vi "Table Test.vi"() -> ()   [LabVIEW 2012]
uses:
  Type/_Table Type.ctl
  Type/_RT Command.ctl
  Configuration/_Global Configuration.vi
panel:
  out "Max Index New":i32
  out "Max Diff New":i32
  out "Current step":i32
  in  "Start":bool
  in  "Table Type":T1
  out "Array":i32[][](array[numeric])
  out "Max Index Old":i32
  out "# of Steps":u32
  out "Max Diff Old":i32
  in  "Step Mass":dbl=0.1
  in  "Stop Mass":dbl=100.0
  in  "Start Mass":dbl
  # "New DAC"
  # "Old DAC"
  # "Actual DAC"
  # "Mass (1/100 amu)"
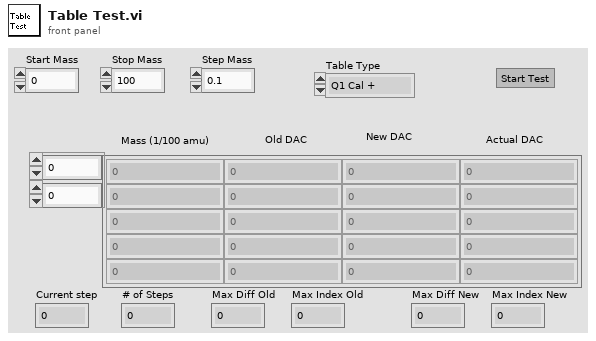
[diagram p1: front panel]
types:
  T1 = typedef "_Table Type.ctl" = enum8{"Q1 Cal +", "Q2 Cal +", "Q1 Cal -", "Q2 Cal -", "Q1 Res Hi +", "Q2 Res Hi +", "Q1 Res Med +", "Q2 Res Med +", "Q1 Res Lo +", "Q2 Res Lo +", "Q1 Res Hi -", "Q2 Res Hi -", "Q1 Res Med -", "Q2 Res Med -", "Q1 Res Lo -", "Q2 Res Lo -"}
  T2 = typedef "_RT Command.ctl" = enum16{"Start", "Stop", "Runtime Update", "Get Data", "Get Info", "Get Status", "Get Param", "Get Config", "Get Table", "Read ADC", "Set Oscillator", "Update Config", "Update Table", "Set All Pol", "Set Pol and DC", "Set Max Mass", "Toggle RP", "Toggle EL", "Set PIC", "Initialize Turbo", "Send Turbo Comm", "Close Turbo", "P1", "P2", "P3", "Send Serial", "Set LC Out", "Get LC In", "Read VAC", "Test Table", "Toggle Power", "Get Startup", "Set Startup", "Get ADC Table", "Set ADC Table", "Get Brief Status", "Get Detail Status", "Auxiliary Update", "Set CC Logics", "Set CC Input Logics", "Ignore Error"}
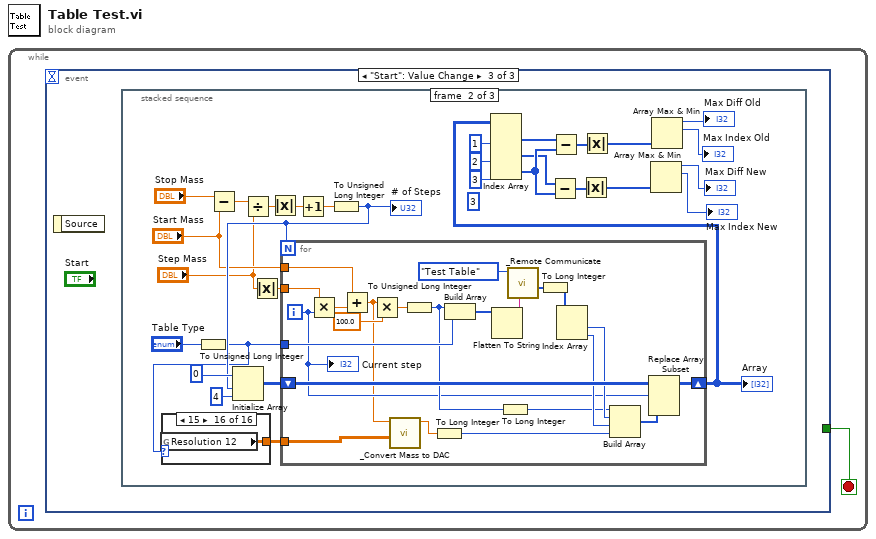
[diagram p0: block diagram]
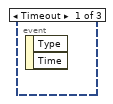
[diagram p2: hidden frame]
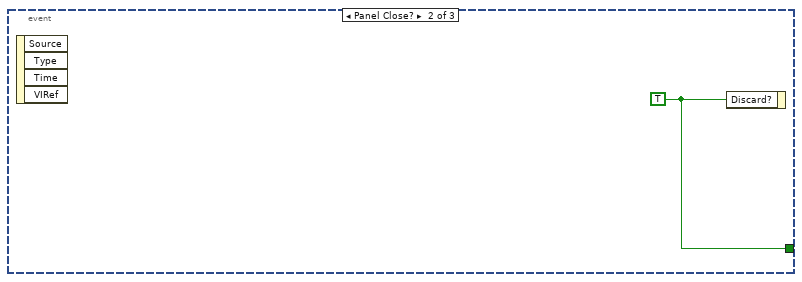
[diagram p3: hidden frame]
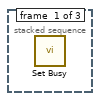
[diagram p4: hidden frame]
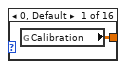
[diagram p5: hidden frame]
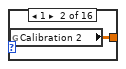
[diagram p6: hidden frame]
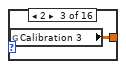
[diagram p7: hidden frame]
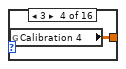
[diagram p8: hidden frame]
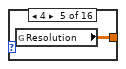
[diagram p9: hidden frame]
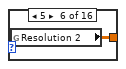
[diagram p10: hidden frame]
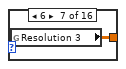
[diagram p11: hidden frame]
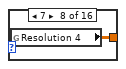
[diagram p12: hidden frame]
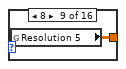
[diagram p13: hidden frame]
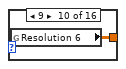
[diagram p14: hidden frame]
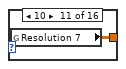
[diagram p15: hidden frame]
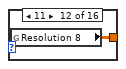
[diagram p16: hidden frame]
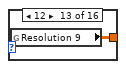
[diagram p17: hidden frame]
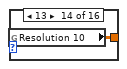
[diagram p18: hidden frame]
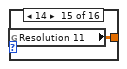
[diagram p19: hidden frame]
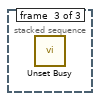
[diagram p20: hidden frame]
diagram:
  n1 = while {
    stop <- w1 stop-if-true
    n2 = event shown="[2] \"Start\": Value Change" {
      selector: _ -> [_ _ _]
      dyn-events: _ -> [_ _ _]
      timeout: _ -> [_ _ _]
      tunnel: [_ w2 _] -> w1
      event Timeout {
        n3 = event-data() -> ()  [unwired: 3 out]
      }
      event Panel Close? {
        w2 = TRUE ("Discard?")
        n4 = event-data() -> ()  [unwired: 5 out]
        n5 = event-data("Discard?"=w2) -> ()  [unwired: 1 in, 1 out]
      }
      event "Start": Value Change {
        n6 = event-data() -> ()  [unwired: 2 out]
        n7 = stacked-sequence {
          frame #0 {
            n8 = call <vilib>:"Set Busy.vi"() -> ()  [unwired: 4 in, 8 out]
          }
          frame #1 {
            (unwired) 3 ("disabled index (col)")
            n9 = To Unsigned Long Integer(number="Table Type") -> (unsigned 32bit integer=w16:u32)
            n10 = case shown="15" w16 {
              tunnel: [w33 w34 w35 w36 w37 w38 w39 w40 w41 w42 w43 w44 w45 w46 w47 w48] -> w15
              frame 0, Default {
                n11 = global read "_Global Configuration.vi" "Calibration"() -> (w33:dbl[][])
              }
              frame 1 {
                n12 = global read "_Global Configuration.vi" "Calibration 2"() -> (w34:dbl[][])
              }
              frame 2 {
                n13 = global read "_Global Configuration.vi" "Calibration 3"() -> (w35:dbl[][])
              }
              frame 3 {
                n14 = global read "_Global Configuration.vi" "Calibration 4"() -> (w36:dbl[][])
              }
              frame 4 {
                n15 = global read "_Global Configuration.vi" "Resolution"() -> (w37:dbl[][])
              }
              frame 5 {
                n16 = global read "_Global Configuration.vi" "Resolution 2"() -> (w38:dbl[][])
              }
              frame 6 {
                n17 = global read "_Global Configuration.vi" "Resolution 3"() -> (w39:dbl[][])
              }
              frame 7 {
                n18 = global read "_Global Configuration.vi" "Resolution 4"() -> (w40:dbl[][])
              }
              frame 8 {
                n19 = global read "_Global Configuration.vi" "Resolution 5"() -> (w41:dbl[][])
              }
              frame 9 {
                n20 = global read "_Global Configuration.vi" "Resolution 6"() -> (w42:dbl[][])
              }
              frame 10 {
                n21 = global read "_Global Configuration.vi" "Resolution 7"() -> (w43:dbl[][])
              }
              frame 11 {
                n22 = global read "_Global Configuration.vi" "Resolution 8"() -> (w44:dbl[][])
              }
              frame 12 {
                n23 = global read "_Global Configuration.vi" "Resolution 9"() -> (w45:dbl[][])
              }
              frame 13 {
                n24 = global read "_Global Configuration.vi" "Resolution 10"() -> (w46:dbl[][])
              }
              frame 14 {
                n25 = global read "_Global Configuration.vi" "Resolution 11"() -> (w47:dbl[][])
              }
              frame 15 {
                n26 = global read "_Global Configuration.vi" "Resolution 12"() -> (w48:dbl[][])
              }
            }
            n27 = Subtract(x="Stop Mass", y="Start Mass") -> (x-y=w31:dbl)
            n28 = Divide(x=w31, y="Step Mass") -> (x/y=w29:dbl)
            n29 = Absolute Value(x="Step Mass") -> (abs(x)=w21:dbl)
            n30 = Absolute Value(x=w29) -> (abs(x)=w30:dbl)
            n31 = Increment(x=w30) -> (x+1=w28:dbl)
            n32 = To Unsigned Long Integer(number=w28) -> (unsigned 32bit integer=w26:u32)
            "# of Steps" <- w26
            n33 = Initialize Array(0, w26, 4 ("dimension size")) -> (w24:i32[][])
            n34 = for {
              N: w26 -> [_]
              shift-right: [w61] -> w19
              shift-left: w24 -> [w62]
              tunnel: "Start Mass" -> [w69]
              tunnel: w21 -> [w71]
              tunnel: w16 -> [w67]
              tunnel: w15 -> [w53]
              i -> [w56]
              n35 = Multiply(x=w71, y=w56) -> (x*y=w70:dbl)
              n36 = Add(x=w69, y=w70) -> (x+y=w54:dbl)
              n37 = Multiply(x=w54, y=100.0) -> (x*y=w55:dbl)
              n38 = call "_Convert Mass to DAC.vi"("Calibration Table"=w53, "Mass"=w54) -> ("DAC Value"=w52:dbl)  [unwired: 2 in, 3 out]
              n39 = To Unsigned Long Integer(number=w55) -> (unsigned 32bit integer=w60:u32)
              n40 = To Long Integer(number=w52) -> (32bit integer=w51:i32)
              n41 = Build Array(w60, w67) -> (w66:u32[])
              n42 = Flatten To String(anything=w66) -> (data string=w65:string)  [unwired: 1 in, 4 out]
              n43 = To Long Integer(number=w60) -> (32bit integer=w50:i32)
              n44 = call "_Remote Communicate.vi"("String"=w65, "Command"=_RT_Command."Test Table") -> ("Data Array"=w63:i32[])  [unwired: 4 in, 3 out]
              n45 = To Long Integer(number=w63) -> (32bit integer=w49:i32[])
              n46 = Index Array(array=w49) -> (element #1=w59:i32, element #2=w58:i32)  [unwired: 2 in]
              n47 = Build Array(w50, w59, w58, w51) -> (w57:i32[])
              n48 = Replace Array Subset(array=w62, new element=w57, index (row)=w56) -> (w61:i32[][])  [unwired: 1 in]
              "Current step" <- w56
            }
            "Array" <- w19
            n49 = Index Array(array=w19, index (col) #1=1 ("disabled index (col)"), index (col) #2=2 ("index (col)"), index (col) #3=3 ("index (col)")) -> (element #1=w11:i32[], element #2=w5:i32[], element #3=w6:i32[])  [unwired: 3 in]
            n50 = Subtract(x=w5, y=w6) -> (x-y=w7:i32[])
            n51 = Subtract(x=w11, y=w6) -> (x-y=w10:i32[])
            n52 = Absolute Value(x=w7) -> (abs(x)=w8:i32[])
            n53 = Absolute Value(x=w10) -> (abs(x)=w9:i32[])
            n54 = Array Max & Min(array=w8) -> (max value=→"Max Diff New":i32, max index (indices)=→"Max Index New":i32)  [unwired: 2 out]
            n55 = Array Max & Min(array=w9) -> (max value=→"Max Diff Old":i32, max index (indices)=→"Max Index Old":i32)  [unwired: 2 out]
          }
          frame #2 {
            n56 = call <vilib>:"Unset Busy.vi"() -> ()  [unwired: 2 in, 10 out]
          }
        }
      }
    }
  }
